vi "Test SetCursor.vi"() -> ()   [LabVIEW 2014, in "Arduino LiquidCrystal Wrapper.lvlib"]
uses:
  Arduino LiquidCrystal Wrapper.lvlib
panel:
  out "Error Out":errorcluster
  in  "Error In":errorcluster
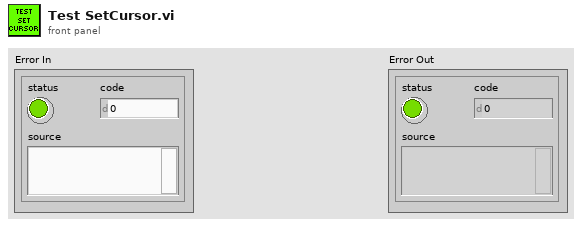
[diagram p1: front panel]
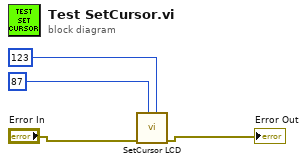
[diagram p0: block diagram]
diagram:
  n1 = call "SetCursor LCD.vi"("row"=u8 123 ("rows"), "col"=u8 87 ("cols"), "Error In"="Error In") -> ("Error Out"=→"Error Out":errorcluster)  [unwired: 8 in]
